vi "init_control_clusterSD.vi"(1 "bounds":T2, 2 "error in (no error)":errorcluster, 3 "references":T1) -> (0 "main cluster":T3={"Experiments groups"=[], "Kinetics"=[], "Spectrum"=[], "GRAPH EXPERIMENTAL DATA"=[], "kinetics plot names"=[], "spectra plot names"=[], "group"=0, "exp selected"=0, "# exp"=0, "error out"={"status"=FALSE, "code"=0, "source"=""}, "FromToWave"={"FromWave"=0.0, "ToWave"=0.0}, "GRAPH EXPERIMENTAL DATA ref"=refnum, "timedelays"=[0.0, 0.0, 0.0, 0.0, 0.0, 0.0, 0.0, 0.06019061100911815, 0.0521779104562645, 0.045231877429679615, 0.03921051490799832, 0.033990728811568754, 0.029465811603150715, 0.025543260876973825, 0.02214288834180205, 0.01919518054014414, 0.016639877791965713, 0.014424742312398925, 0.012504490320209958, 0.010839866306230088, 0.009396840537117498, 0.008145913389103785, 0.00706151229029317, 0.006121468943269439, 0.005306566140927374, 0.004600144911132549, 0.003987763959109073, 0.0034569044455719407, 0.00299671406541447, 0.0025977851951783253, 0.0022519625739982996, 0.00195217658646366, 0.0016922987392150965, 0.0014670163768006634, 0.0012717240756200802, 0.0011024294957352762, 0.0009556717658856477, 0.0008284507332614981, 0.0007181656316962257, 0.0006225619144775864, 0.0005396851648867825, 0.00046784114226338394, 0.0004055611468220084, 0.0003515719951773376, 0.00030476999279031153, 0.00026419837125694315, 0.00022902772919263772, 0.0001985390768670671, 0.0001721091379728629, 0.00014919760805372974, 0.00012933610911736794], "wavelengths"=[0.0, 0.0, 0.0, 0.0, 0.0, 0.0, 0.0, 0.06019061100911815, 0.0521779104562645, 0.045231877429679615, 0.03921051490799832, 0.033990728811568754, 0.029465811603150715, 0.025543260876973825, 0.02214288834180205, 0.01919518054014414, 0.016639877791965713, 0.014424742312398925, 0.012504490320209958, 0.010839866306230088, 0.009396840537117498, 0.008145913389103785, 0.00706151229029317, 0.006121468943269439, 0.005306566140927374, 0.004600144911132549, 0.003987763959109073, 0.0034569044455719407, 0.00299671406541447, 0.0025977851951783253, 0.0022519625739982996, 0.00195217658646366, 0.0016922987392150965, 0.0014670163768006634, 0.0012717240756200802, 0.0011024294957352762, 0.0009556717658856477, 0.0008284507332614981, 0.0007181656316962257, 0.0006225619144775864, 0.0005396851648867825, 0.00046784114226338394, 0.0004055611468220084, 0.0003515719951773376, 0.00030476999279031153, 0.00026419837125694315, 0.00022902772919263772, 0.0001985390768670671, 0.0001721091379728629, 0.00014919760805372974, 0.00012933610911736794], "Experiment"=refnum, "Commentaires exp"=refnum, "FromToDelay"={"FromDelay"=0.0, "ToDelay"=0.0}})   [LabVIEW 2015]
uses:
  controls/control-cluster.ctl
  Classes/Experiments_group.lvclass
  Classes/Experiment.lvclass
  globalVarSD.vi
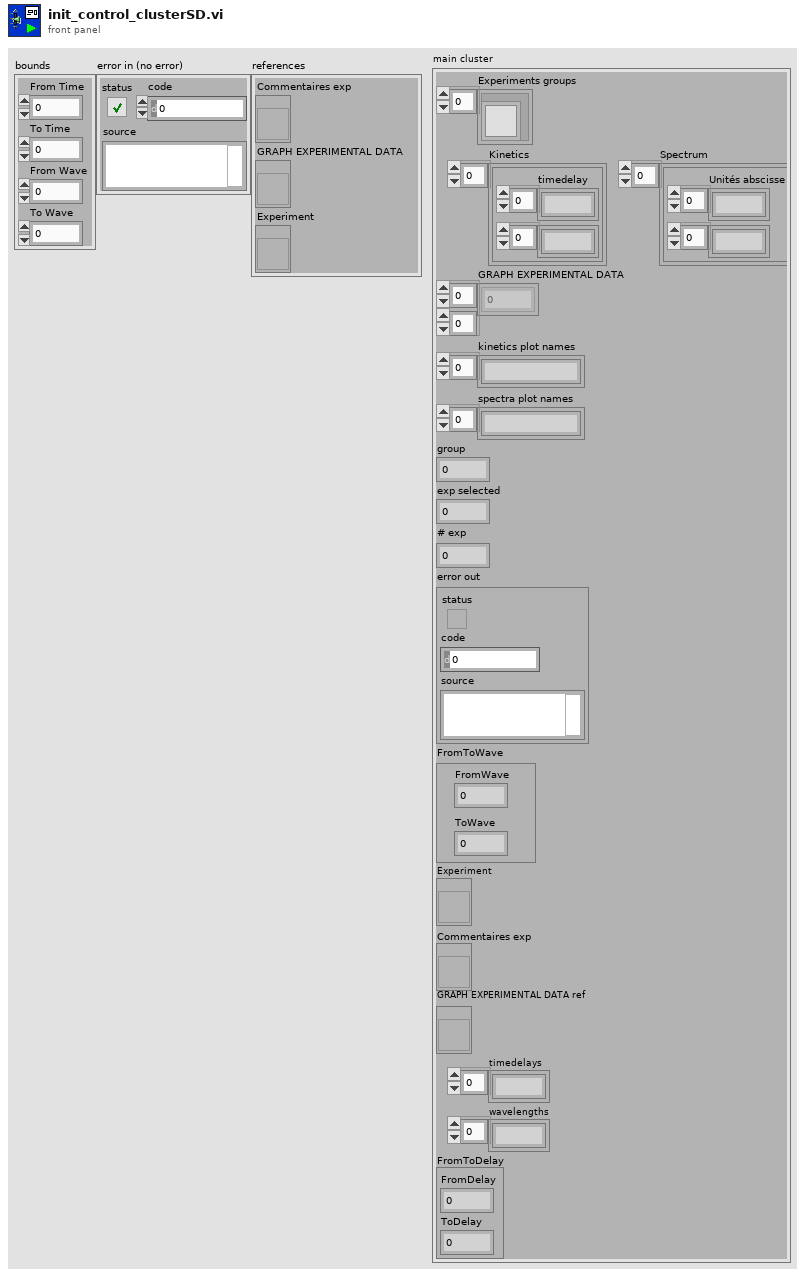
[diagram p1: front panel]
types:
  T1 = cluster{"Commentaires exp":refnum<vi>, "GRAPH EXPERIMENTAL DATA":refnum<vi>, "Experiment":refnum<vi>}
  T2 = cluster{"From Time":dbl, "To Time":dbl, "From Wave":dbl, "To Wave":dbl}
  T3 = typedef "control-cluster.ctl" = cluster{"Experiments groups":refnum<class "Experiments_group.lvclass">[], "Kinetics":cluster{"timedelay":dbl[], dbl[]}[], "Spectrum":cluster{"Unités abscisse":dbl[], dbl[]}[], "GRAPH EXPERIMENTAL DATA":dbl[][], "kinetics plot names":string[], "spectra plot names":string[], "group":i32, "exp selected":i32, "# exp":i32, "error out":errorcluster, "FromToWave":cluster{"FromWave":dbl, "ToWave":dbl}, "GRAPH EXPERIMENTAL DATA ref":refnum<vi>, "timedelays":dbl[], "wavelengths":dbl[], "Experiment":refnum<vi>, "Commentaires exp":refnum<vi>, "FromToDelay":cluster{"FromDelay":dbl, "ToDelay":dbl}}
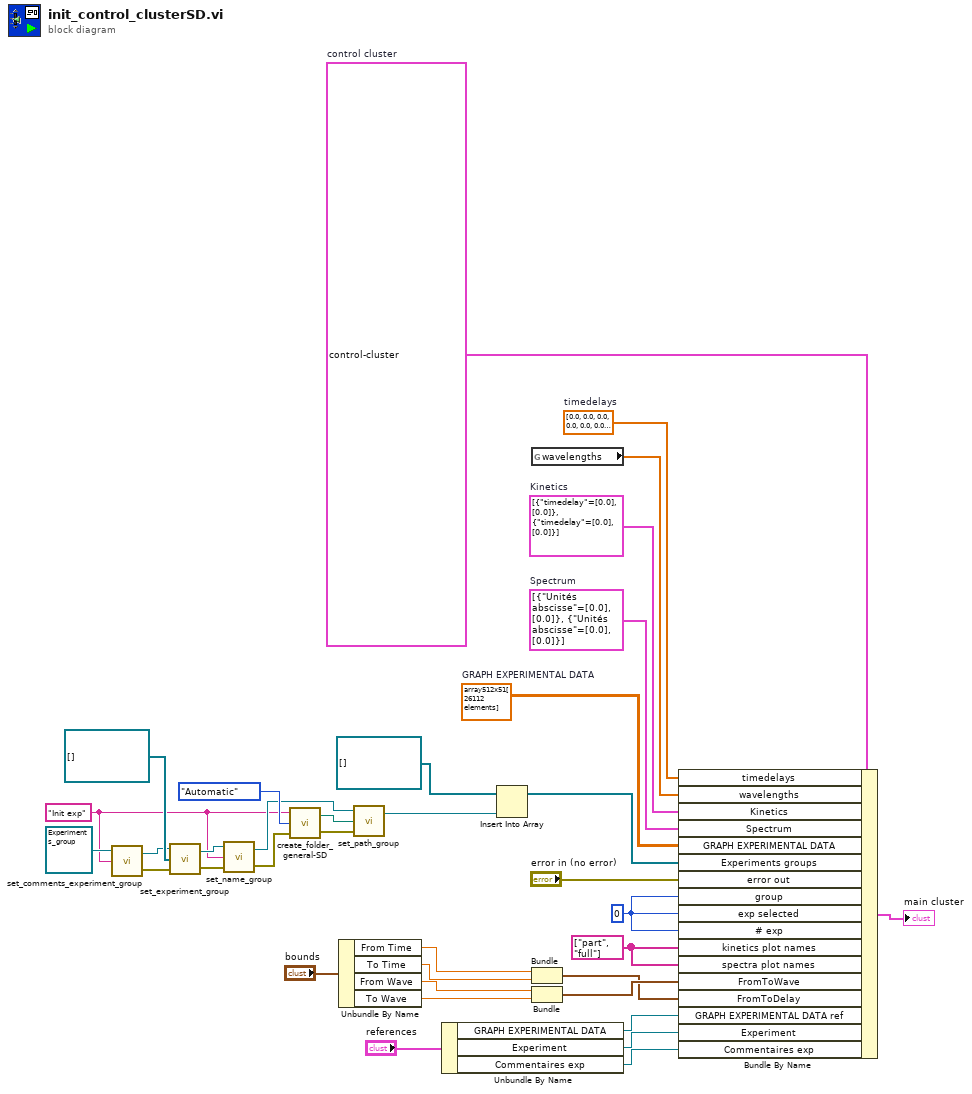
[diagram p0: block diagram]
diagram:
  w10 = "Init exp" ("Comments")
  w4 = T3 {"Experiments groups"=[], "Kinetics"=[], "Spectrum"=[], "GRAPH EXPERIMENTAL DATA"=[], "kinetics plot names"=[], "spectra plot names"=[], "group"=0, "exp selected"=0, "# exp"=0, "error out"={"status"=FALSE, "code"=0, "source"=""}, "FromToWave"={"FromWave"=0.0, "ToWave"=0.0}, "GRAPH EXPERIMENTAL DATA ref"=refnum, "timedelays"=[0.0, 0.0, 0.0, 0.0, 0.0, 0.0, 0.0, 0.06019061100911815, 0.0521779104562645, 0.045231877429679615, 0.03921051490799832, 0.033990728811568754, 0.029465811603150715, 0.025543260876973825, 0.02214288834180205, 0.01919518054014414, 0.016639877791965713, 0.014424742312398925, 0.012504490320209958, 0.010839866306230088, 0.009396840537117498, 0.008145913389103785, 0.00706151229029317, 0.006121468943269439, 0.005306566140927374, 0.004600144911132549, 0.003987763959109073, 0.0034569044455719407, 0.00299671406541447, 0.0025977851951783253, 0.0022519625739982996, 0.00195217658646366, 0.0016922987392150965, 0.0014670163768006634, 0.0012717240756200802, 0.0011024294957352762, 0.0009556717658856477, 0.0008284507332614981, 0.0007181656316962257, 0.0006225619144775864, 0.0005396851648867825, 0.00046784114226338394, 0.0004055611468220084, 0.0003515719951773376, 0.00030476999279031153, 0.00026419837125694315, 0.00022902772919263772, 0.0001985390768670671, 0.0001721091379728629, 0.00014919760805372974, 0.00012933610911736794], "wavelengths"=[0.0, 0.0, 0.0, 0.0, 0.0, 0.0, 0.0, 0.06019061100911815, 0.0521779104562645, 0.045231877429679615, 0.03921051490799832, 0.033990728811568754, 0.029465811603150715, 0.025543260876973825, 0.02214288834180205, 0.01919518054014414, 0.016639877791965713, 0.014424742312398925, 0.012504490320209958, 0.010839866306230088, 0.009396840537117498, 0.008145913389103785, 0.00706151229029317, 0.006121468943269439, 0.005306566140927374, 0.004600144911132549, 0.003987763959109073, 0.0034569044455719407, 0.00299671406541447, 0.0025977851951783253, 0.0022519625739982996, 0.00195217658646366, 0.0016922987392150965, 0.0014670163768006634, 0.0012717240756200802, 0.0011024294957352762, 0.0009556717658856477, 0.0008284507332614981, 0.0007181656316962257, 0.0006225619144775864, 0.0005396851648867825, 0.00046784114226338394, 0.0004055611468220084, 0.0003515719951773376, 0.00030476999279031153, 0.00026419837125694315, 0.00022902772919263772, 0.0001985390768670671, 0.0001721091379728629, 0.00014919760805372974, 0.00012933610911736794], "Experiment"=refnum, "Commentaires exp"=refnum, "FromToDelay"={"FromDelay"=0.0, "ToDelay"=0.0}}  # control cluster
  w8 = dbl[] [0.0, 0.0, 0.0, 0.0, 0.0, 0.0, 0.0, 0.06019061100911815, 0.0521779104562645, 0.045231877429679615, 0.03921051490799832, 0.033990728811568754, 0.029465811603150715, 0.025543260876973825, 0.02214288834180205, 0.01919518054014414, 0.016639877791965713, 0.014424742312398925, 0.012504490320209958, 0.010839866306230088, 0.009396840537117498, 0.008145913389103785, 0.00706151229029317, 0.006121468943269439, 0.005306566140927374, 0.004600144911132549, 0.003987763959109073, 0.0034569044455719407, 0.00299671406541447, 0.0025977851951783253, 0.0022519625739982996, 0.00195217658646366, 0.0016922987392150965, 0.0014670163768006634, 0.0012717240756200802, 0.0011024294957352762, 0.0009556717658856477, 0.0008284507332614981, 0.0007181656316962257, 0.0006225619144775864, 0.0005396851648867825, 0.00046784114226338394, 0.0004055611468220084, 0.0003515719951773376, 0.00030476999279031153, 0.00026419837125694315, 0.00022902772919263772, 0.0001985390768670671, 0.0001721091379728629, 0.00014919760805372974, 0.00012933610911736794]  # timedelays
  w5 = string[] ["part", "full"] ("kinetics plot names")
  w6 = 0 ("exp selected")
  w3 = dbl[][] array512x51[26112 elements]  # GRAPH EXPERIMENTAL DATA
  w1 = cluster{"timedelay":dbl[], dbl[]}[] [{"timedelay"=[0.0], [0.0]}, {"timedelay"=[0.0], [0.0]}]  # Kinetics
  w2 = cluster{"Unités abscisse":dbl[], dbl[]}[] [{"Unités abscisse"=[0.0], [0.0]}, {"Unités abscisse"=[0.0], [0.0]}]  # Spectrum
  n1 = call-dynamic "set_comments_experiment_group.vi"("Comments"=w10, "Experiments_group.lvclass in"=refnum<class "Experiments_group.lvclass"> refnum ("Experiments_group.lvclass")) -> ("error out"=w18:errorcluster, "Experiments_group.lvclass out"=w16:refnum<class "Experiments_group.lvclass">)  [unwired: 1 in]
  n2 = call-dynamic "set_experiment_group.vi"("error in (no error)"=w18, "Experiments"=refnum<class "Experiment.lvclass">[] [] ("Experiment array"), "Experiments_group.lvclass in"=w16) -> ("error out"=w14:errorcluster, "Experiments_group.lvclass out"=w12:refnum<class "Experiments_group.lvclass">)
  n3 = call-dynamic "set_name_group.vi"("error in (no error)"=w14, "Name"=w10, "Experiments_group.lvclass in"=w12) -> ("error out"=w13:errorcluster, "Experiments_group.lvclass out"=w11:refnum<class "Experiments_group.lvclass">)
  n4 = call "create_folder_general-SD.vi"("error in (no error)"=w13, "save Radio Buttons"=enum32{"Automatic", "User-def"}."Automatic", "Name"=w10) -> ("error out"=w20:errorcluster, "appended path"=w21:path)
  n5 = Unbundle By Name("bounds") -> ("From Time"=w27:dbl, "To Time"=w28:dbl, "From Wave"=w29:dbl, "To Wave"=w30:dbl)
  n6 = call-dynamic "set_path_group.vi"("error in (no error)"=w20, "Path"=w21, "Experiments_group.lvclass in"=w11) -> ("Experiments_group.lvclass out"=w15:refnum<class "Experiments_group.lvclass">)  [unwired: 1 out]
  n7 = Unbundle By Name("references") -> ("GRAPH EXPERIMENTAL DATA"=w36:refnum<vi>, "Experiment"=w35:refnum<vi>, "Commentaires exp"=w34:refnum<vi>)
  n8 = Insert Into Array(array=refnum<class "Experiments_group.lvclass">[] [] ("Experiments groups"), new element=w15) -> (w24:refnum<class "Experiments_group.lvclass">[])  [unwired: 1 in]
  n9 = global read "globalVarSD.vi" "wavelengths"() -> (w9:dbl[])
  n10 = Bundle("From Time"=w27, "To Time"=w28) -> (w31:cluster{"From Time":dbl, "To Time":dbl})  [unwired: 1 in]
  n11 = Bundle("From Wave"=w29, "To Wave"=w30) -> (w32:cluster{"From Wave":dbl, "To Wave":dbl})  [unwired: 1 in]
  n12 = Bundle By Name(cluster=w4, "timedelays"=w8, "wavelengths"=w9, "Kinetics"=w1, "Spectrum"=w2, "GRAPH EXPERIMENTAL DATA"=w3, "Experiments groups"=w24, "error out"="error in (no error)", "group"=w6, "exp selected"=w6, "# exp"=w6, "kinetics plot names"=w5, "spectra plot names"=w5, "FromToWave"=w32, "FromToDelay"=w31, "GRAPH EXPERIMENTAL DATA ref"=w36, "Experiment"=w35, "Commentaires exp"=w34) -> (→"main cluster":T3)
